vi "ISO 8601拡張形式で時刻を返す.vi"(7 "UTC形式":bool, 8 "Error In":errorcluster caption="エラー入力", 11 "タイムスタンプ":timestamp) -> (0 "Error Out":errorcluster caption="エラー出力", 3 "日付/時間文字列":string)   [LabVIEW 2018]
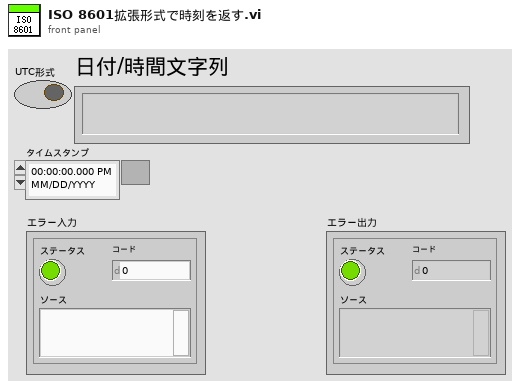
[diagram p1: front panel]
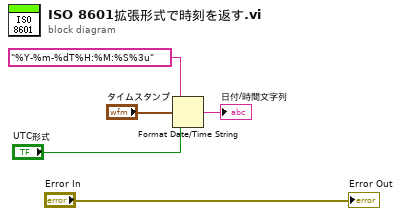
[diagram p0: block diagram]
diagram:
  n1 = Format Date/Time String(time format string (%c)="%Y-%m-%dT%H:%M:%S%3u" ("時間形式文字列（%c）"), seconds (now)="タイムスタンプ", UTC format="UTC形式") -> (date/time string=→"日付/時間文字列":string)
  "Error Out" <- "Error In"
